vi "CodigoBinGrey.vi"() -> ()   [LabVIEW 2021]
panel:
  out "d":bool
  out "c":bool
  out "b":bool
  out "a":bool
  in  "D":bool
  in  "C":bool
  in  "B":bool
  in  "A":bool
  # "Mendoza Meza Manuel Everardo"
  # "Convertidor codigo Binario a codigo Grey"
  # "Binario"
  # "Grey"
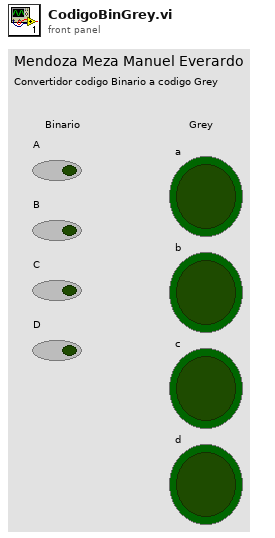
[diagram p1: front panel]
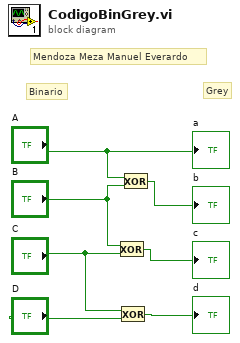
[diagram p0: block diagram]
diagram:
  # "Grey"
  # "Binario"
  # "Mendoza Meza Manuel Everardo"
  n1 = Exclusive Or(1:"C", 2:"B") -> (0:→"c":bool)
  n2 = Exclusive Or(1:"D", 2:"C") -> (0:→"d":bool)
  n3 = Exclusive Or(1:"B", 2:"A") -> (0:→"b":bool)
  "a" <- "A"
